vi "1553B_帧解析.vi"(11 "数组":u8[](array[numeric])) -> (3 "帧数据":T1)   [LabVIEW 2012]
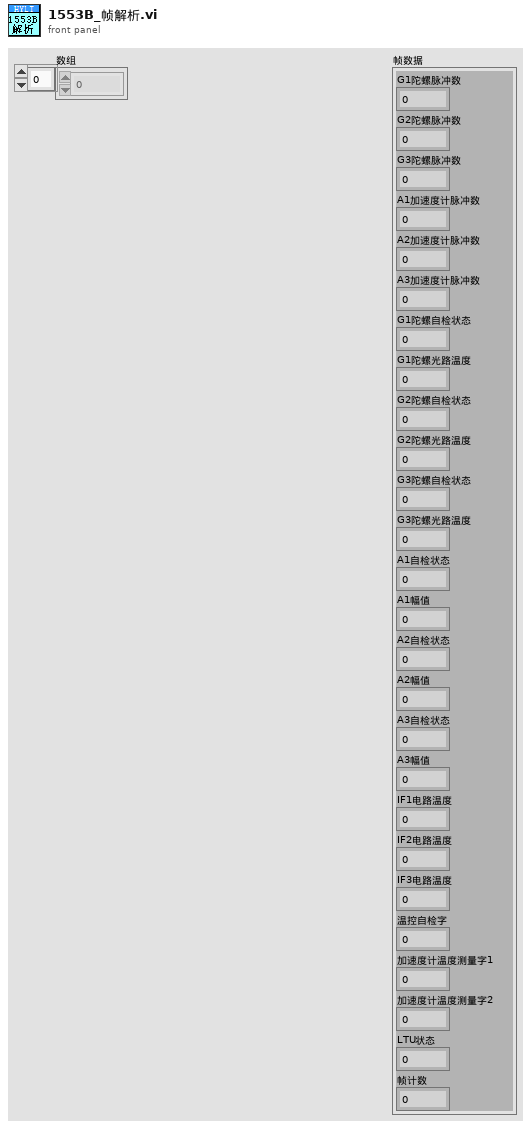
[diagram p1: front panel]
types:
  T1 = cluster{"G1陀螺脉冲数":u32, "G2陀螺脉冲数":u32, "G3陀螺脉冲数":u32, "A1加速度计脉冲数":u32, "A2加速度计脉冲数":u32, "A3加速度计脉冲数":u32, "G1陀螺自检状态":u8, "G1陀螺光路温度":u8, "G2陀螺自检状态":u8, "G2陀螺光路温度":u8, "G3陀螺自检状态":u8, "G3陀螺光路温度":u8, "A1自检状态":u8, "A1幅值":u8, "A2自检状态":u8, "A2幅值":u8, "A3自检状态":u8, "A3幅值":u8, "IF1电路温度":u8, "IF2电路温度":u8, "IF3电路温度":u8, "温控自检字":u8, "加速度计温度测量字1":u32, "加速度计温度测量字2":u32, "LTU状态":u8, "帧计数":u8}
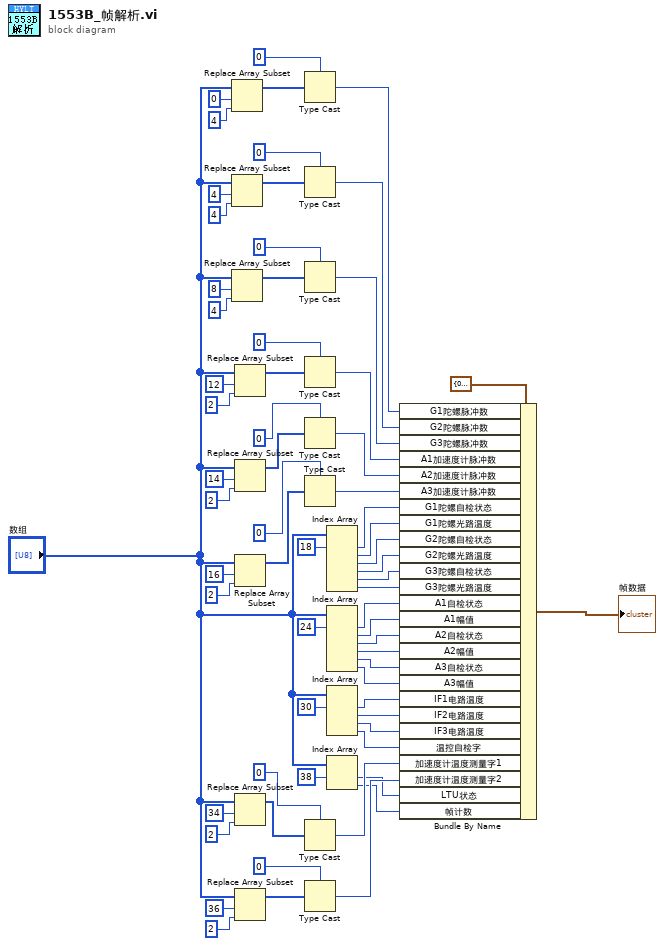
[diagram p0: block diagram]
diagram:
  n1 = Replace Array Subset(array="数组", new element=u8 4 ("新元素/子数组"), index=0 ("索引")) -> (w63:u8[])
  n2 = Replace Array Subset(array="数组", new element=u8 4 ("新元素/子数组"), index=4 ("索引")) -> (w60:u8[])
  n3 = Replace Array Subset(array="数组", new element=u8 4 ("新元素/子数组"), index=8 ("索引")) -> (w55:u8[])
  n4 = Replace Array Subset(array="数组", new element=u8 2 ("新元素/子数组"), index=12 ("索引")) -> (w52:u8[])
  n5 = Replace Array Subset(array="数组", new element=u8 2 ("新元素/子数组"), index=14 ("索引")) -> (w47:u8[])
  n6 = Replace Array Subset(array="数组", new element=u8 2 ("新元素/子数组"), index=16 ("索引")) -> (w44:u8[])
  n7 = Replace Array Subset(array="数组", new element=u8 2 ("新元素/子数组"), index=34 ("索引")) -> (w34:u8[])
  n8 = Replace Array Subset(array="数组", new element=u8 2 ("新元素/子数组"), index=36 ("索引")) -> (w37:u8[])
  n9 = Type Cast(type=u32 0, x=w63) -> (*(type *) &x=w28:u32)
  n10 = Type Cast(type=u32 0, x=w60) -> (*(type *) &x=w27:u32)
  n11 = Type Cast(type=u32 0, x=w55) -> (*(type *) &x=w26:u32)
  n12 = Type Cast(type=u32 0, x=w52) -> (*(type *) &x=w25:u32)
  n13 = Type Cast(type=u32 0, x=w47) -> (*(type *) &x=w24:u32)
  n14 = Type Cast(type=u32 0, x=w44) -> (*(type *) &x=w23:u32)
  n15 = Type Cast(type=u32 0, x=w34) -> (*(type *) &x=w6:u32)
  n16 = Type Cast(type=u32 0, x=w37) -> (*(type *) &x=w5:u32)
  n17 = Index Array(array="数组", index #1=18 ("索引")) -> (element #1=w22:u8, element #2=w21:u8, element #3=w20:u8, element #4=w19:u8, element #5=w18:u8, element #6=w17:u8)  [unwired: 5 in]
  n18 = Index Array(array="数组", index #1=24 ("索引")) -> (element #1=w16:u8, element #2=w15:u8, element #3=w14:u8, element #4=w13:u8, element #5=w12:u8, element #6=w11:u8)  [unwired: 5 in]
  n19 = Index Array(array="数组", index #1=30 ("索引")) -> (element #1=w10:u8, element #2=w9:u8, element #3=w8:u8, element #4=w7:u8)  [unwired: 3 in]
  n20 = Index Array(array="数组", index #1=38 ("索引")) -> (element #1=w4:u8, element #2=w3:u8)  [unwired: 1 in]
  n21 = Bundle By Name(cluster=T1 {"G1陀螺脉冲数"=0, "G2陀螺脉冲数"=0, "G3陀螺脉冲数"=0, "A1加速度计脉冲数"=0, "A2加速度计脉冲数"=0, "A3加速度计脉冲数"=0, "G1陀螺自检状态"=0, "G1陀螺光路温度"=0, "G2陀螺自检状态"=0, "G2陀螺光路温度"=0, "G3陀螺自检状态"=0, "G3陀螺光路温度"=0, "A1自检状态"=0, "A1幅值"=0, "A2自检状态"=0, "A2幅值"=0, "A3自检状态"=0, "A3幅值"=0, "IF1电路温度"=0, "IF2电路温度"=0, "IF3电路温度"=0, "温控自检字"=0, "加速度计温度测量字1"=0, "加速度计温度测量字2"=0, "LTU状态"=0, "帧计数"=0} ("输入簇"), "G1陀螺脉冲数"=w28, "G2陀螺脉冲数"=w27, "G3陀螺脉冲数"=w26, "A1加速度计脉冲数"=w25, "A2加速度计脉冲数"=w24, "A3加速度计脉冲数"=w23, "G1陀螺自检状态"=w22, "G1陀螺光路温度"=w21, "G2陀螺自检状态"=w20, "G2陀螺光路温度"=w19, "G3陀螺自检状态"=w18, "G3陀螺光路温度"=w17, "A1自检状态"=w16, "A1幅值"=w15, "A2自检状态"=w14, "A2幅值"=w13, "A3自检状态"=w12, "A3幅值"=w11, "IF1电路温度"=w10, "IF2电路温度"=w9, "IF3电路温度"=w8, "温控自检字"=w7, "加速度计温度测量字1"=w6, "加速度计温度测量字2"=w5, "LTU状态"=w4, "帧计数"=w3) -> (→"帧数据":T1)
